vi "фильтр 1.vi"(0 "Image In":T1, 1 "Image Dst":T1, 7 "error in":errorcluster, 8 "Truncation Frequency %":sgl=10.0 format="%.2f") -> (20 "Image Out":T1, 27 "error out":errorcluster)   [LabVIEW 2011]
doc: "Creates, edits, and runs vision algorithms using NI Vision Assistant.\n\nWhen you place this Express VI on the block diagram, NI Vision Assistant launches. Create an algorithm using the Vision Assistant processing functions. After you create an algorithm, you can select the controls and indicators that you want to be able to programmatically set in LabVIEW. Double-click the Vision Assistant Express VI to edit the algorithm."
uses:
  <vilib>/vision/Image Controls.llb/IMAQ Image.ctl
  <vilib>/vision/NI_Vision_Development_Module.lvlib
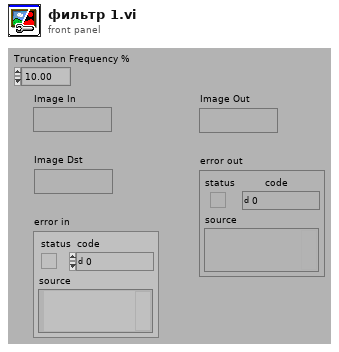
[diagram p1: front panel]
types:
  T1 = typedef "IMAQ Image.ctl" = refnum<image>
  T2 = typedef "Image Type" = u32
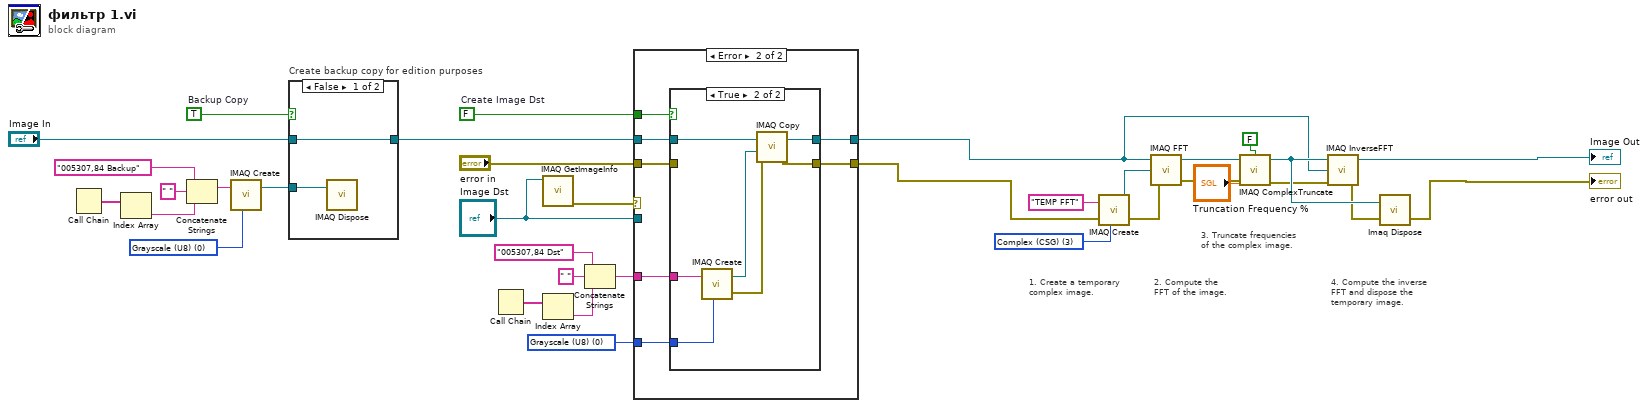
[diagram p0: block diagram]
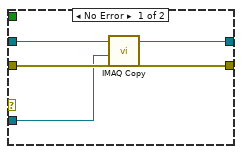
[diagram p2: hidden frame]
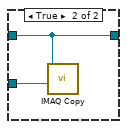
[diagram p4: hidden frame]
diagram:
  w3 = T2 3 items=["Grayscale (U8)", "Grayscale (I16)", "Grayscale (SGL)", "Complex (CSG)", "RGB (U32)", "HSL (U32)", "RGB (U64)", "Grayscale (U16)"] ("Image Type")
  w15 = T2 0 items=["Grayscale (U8)", "Grayscale (I16)", "Grayscale (SGL)", "Complex (CSG)", "RGB (U32)", "HSL (U32)", "RGB (U64)", "Grayscale (U16)"] ("Image Dst Type")
  w16 = T2 0 items=["Grayscale (U8)", "Grayscale (I16)", "Grayscale (SGL)", "Complex (CSG)", "RGB (U32)", "HSL (U32)", "RGB (U64)", "Grayscale (U16)"] ("Image Type")
  w35 = TRUE  # Backup Copy
  w28 = FALSE  # Create Image Dst
  # "4. Compute the inverse\nFFT and dispose the\ntemporary image."
  # "3. Truncate frequencies\nof the complex image."
  # "2. Compute the\nFFT of the image."
  # "1. Create a temporary\ncomplex image."
  n1 = Call Chain() -> (call chain=w22:string[])
  n2 = Index Array(array=w22) -> (element=w21:string)  [unwired: 1 in]
  n3 = Concatenate Strings("005307,84 Backup" ("Backup Image Name"), " ", w21) -> (w18:string)
  n4 = call "IMAQ Create"("Image Name"=w18, "Image Type"=w16) -> ("New Image"=w17:T1)  [unwired: 2 in, 2 out]
  n5 = case "Create backup copy for edition purposes" shown="False" w35 {
    tunnel: [w37 w39] -> w31
    tunnel: "Image In" -> [w37 w39]
    tunnel: w17 -> [w36 w38]
    frame False {
      n6 = call "IMAQ Dispose"("Image"=w36) -> ()  [unwired: 2 in, 4 out]
    }
    frame True {
      n7 = call "IMAQ Copy"("Image Dst"=w38, "Image Src"=w39) -> ()  [unwired: 1 in, 5 out]
    }
  }
  n8 = Call Chain() -> (call chain=w27:string[])
  n9 = call "IMAQ GetImageInfo"("Image"="Image Dst") -> ("error out"=w33:errorcluster)  [unwired: 1 in, 9 out]
  n10 = Index Array(array=w27) -> (element=w25:string)  [unwired: 1 in]
  n11 = Concatenate Strings("005307,84 Dst" ("Image Dst Name"), " ", w25) -> (w23:string)
  n12 = case shown="Error" w33 {
    tunnel: [w44 w48] -> w5
    tunnel: [w43 w47] -> w29
    tunnel: w31 -> [w42 w49]
    tunnel: "error in" -> [w41 w45]
    tunnel: "Image Dst" -> [w40 _]
    tunnel: w23 -> [_ w51]
    tunnel: w15 -> [_ w50]
    tunnel: w28 -> [_ w46]
    frame No Error {
      n13 = call "IMAQ Copy"("error in (no error)"=w41, "Image Dst"=w40, "Image Src"=w42) -> ("error out"=w43:errorcluster, "Image Dst Out"=w44:T1)  [unwired: 3 out]
    }
    frame Error {
      n14 = case shown="True" w46 {
        tunnel: w51 -> [_ w60]
        tunnel: w50 -> [_ w59]
        tunnel: w49 -> [w53 w57]
        tunnel: [w53 w56] -> w48
        tunnel: [w52 w55] -> w47
        tunnel: w45 -> [w52 _]
        frame False {
        }
        frame True {
          n15 = call "IMAQ Create"("Image Name"=w60, "Image Type"=w59) -> ("New Image"=w58:T1, "error out"=w54:errorcluster)  [unwired: 2 in, 1 out]
          n16 = call "IMAQ Copy"("error in (no error)"=w54, "Image Dst"=w58, "Image Src"=w57) -> ("error out"=w55:errorcluster, "Image Dst Out"=w56:T1)  [unwired: 3 out]
        }
      }
    }
  }
  n17 = call "IMAQ Create"("Image Name"="TEMP FFT", "Image Type"=w3, "error in (no error)"=w29) -> ("New Image"=w13:T1, "error out"=w6:errorcluster)  [unwired: 1 in, 1 out]
  n18 = call "IMAQ FFT"("error in (no error)"=w6, "Image Dst"=w13, "Image Src"=w5) -> ("error out"=w11:errorcluster, "Image Dst Out"=w12:T1)  [unwired: 1 out]
  n19 = call "IMAQ ComplexTruncate"("error in (no error)"=w11, "Truncation Frequency %"="Truncation Frequency %", "Image Src"=w12, "Low pass/High pass (Low pass)"=FALSE) -> ("error out"=w9:errorcluster, "Image Dst Out"=w10:T1)  [unwired: 1 in, 2 out]
  n20 = call "IMAQ InverseFFT"("error in (no error)"=w9, "Image Dst"=w5, "Image Src"=w10) -> ("error out"=w8:errorcluster, "Image Dst Out"=→"Image Out":T1)  [unwired: 1 out]
  n21 = call "Imaq Dispose"("Image"=w10, "error in (no error)"=w8) -> ("error out"=→"error out":errorcluster)  [unwired: 1 in, 3 out]
